vi "SVT Get Octave Value (N Ch).vi"(0 "octave spectra":T5(array[cluster]) {"band power" format="%.2f"; "nominal frequencies [Hz]" format="%.2f"}, 5 "frequency [Hz]":dbl=1000.0 format="%.2f", 9 "octave info":T1[](array[typedef]) {"engineering units" items=["custom..."=0, "V"=1, "A"=21, "C"=30, "pC"=31, "s"=32, "-"=29, "Pa"=2, "N"=20, "g"=3, "m/s^2"=4, "m/s"=5, "m"=6, "mm/s"=12, "mm"=13, "micron/s"=14, "micron"=15, "in/s^2"=7, "in/s"=8, "in"=9, "mil/s"=10, "mil"=11, "rad/s^2"=16, "rad/s"=17, "rad"=18, "deg/s^2"=26, "deg/s"=27, "deg"=28, "RPM"=22, "cycle/s^2"=23, "Hz"=24, "cycle"=25, "strain"=19]; "dB reference" format="%.2e"; "weighting filter" items=["Linear", "A-weighting", "B-weighting", "C-weighting", "ITU-R 468-4", "Dolby", "CCITT", "C-message", "Wb", "Wc", "Wd", "We", "Wf", "Wh", "Wj", "Wk", "Wm", "AES17 20 kHz lowpass", "AES17 40 kHz lowpass", "AES17 20 kHz highpass", "AES17 40 kHz highpass"]}, 11 "error in (no error)":errorcluster) -> (4 "band power values":dbl[](array[numeric]), 6 "unit labels":string[](array[string]), 8 "actual nominal frequencies [Hz]":dbl[](array[numeric]), 15 "error out":errorcluster)   [LabVIEW 2017, in "SoundVib_Octave_2014 standard.lvlib"]
doc: "Extracts the band power value of the <B>octave spectrum</B> at the specified input frequency. Finds the octave band that corresponds to the input frequency if the input frequency does not exactly coincide with a nominal frequency. Wire data to the <B>octave spectrum</B> input to determine the polymorphic instance to use or manually select the instance."
uses:
  <vilib>/addons/Sound and Vibration/svt_Octave/SoundVib_Octave_2014 standard.lvlib
  <vilib>/addons/_NISVFA/_Shared subVIs/Controls/svc_Octave Info.ctl
  <vilib>/addons/_NISVFA/_Shared subVIs/Controls/svc_Octave Standard.ctl
  <vilib>/addons/_NISVFA/_Shared subVIs/Controls/svc_Weighting Filter Text Ring.ctl
  <vilib>/addons/_NISVFA/_Shared subVIs/Controls/svc_Engineering Units Text Ring.ctl
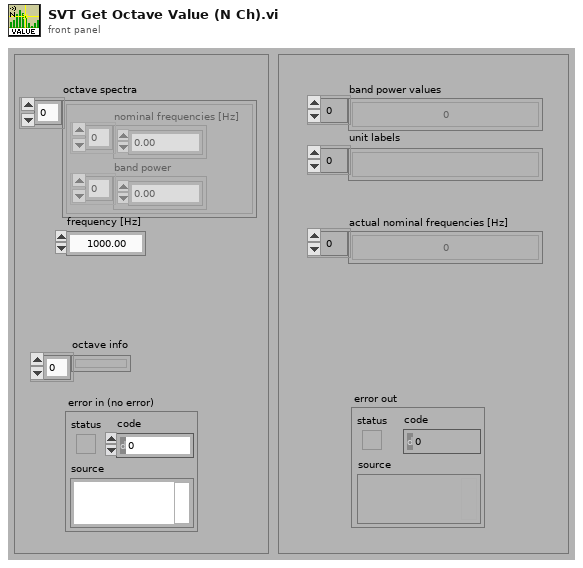
[diagram p1: front panel]
types:
  T1 = typedef "svc_Octave Info.ctl" = cluster{"standard":T2, "bandwidth":enum16{"1 octave", "1/3 octave", "1/6 octave", "1/12 octave", "1/24 octave"}, "low band":i32, "high band":i32, "weighting filter":T3, "dB reference":dbl, "dB On":bool, "unit label":string, "channel name":string, "description":string, "engineering units":T4, "custom label":string, "spectrum type":enum16{"power", "magnitude"}, "spectral density":bool, "filters settled":bool}
  T2 = typedef "svc_Octave Standard.ctl" = enum16{"ANSI S1.11", "IEC 61260"}
  T3 = typedef "svc_Weighting Filter Text Ring.ctl" = u16
  T4 = typedef "svc_Engineering Units Text Ring.ctl" = u16
  T5 = cluster{"nominal frequencies [Hz]":dbl[], "band power":dbl[]}[]
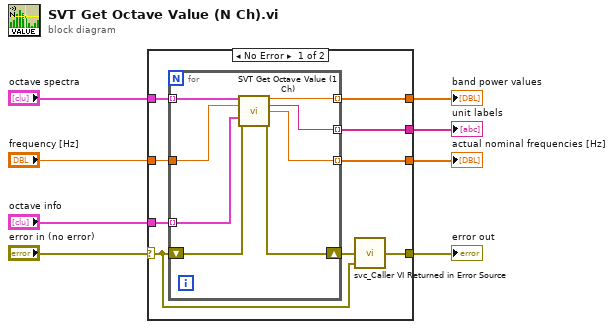
[diagram p0: block diagram]
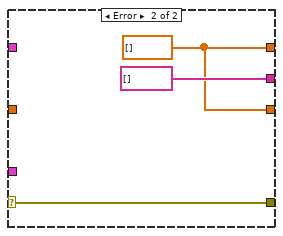
[diagram p2: hidden frame]
diagram:
  n1 = case shown="No Error" "error in (no error)" {
    tunnel: [w17 w28] -> w8
    tunnel: "octave info" -> [w15 _]
    tunnel: "octave spectra" -> [w16 _]
    tunnel: [w14 w26] -> w5
    tunnel: [w13 string[] []] -> w3
    tunnel: "frequency [Hz]" -> [w12 _]
    tunnel: [w11 w26] -> w2
    selector: "error in (no error)" -> [w9 w28]
    frame No Error {
      n2 = for {
        tunnel: w16 -> [w23] mode=indexing
        tunnel: w15 -> [w22] mode=indexing
        tunnel: [w21] -> w14 mode=indexing
        tunnel: [w20] -> w13 mode=indexing
        tunnel: w12 -> [w18]
        tunnel: [w19] -> w11 mode=indexing
        shift-right: [w24] -> w10
        shift-left: w9 -> [w25]
        n3 = call <vilib>:"SVT Get Octave Value (1 Ch).vi"("octave spectrum"=w23, "frequency [Hz]"=w18, "octave info"=w22, "error in (no error)"=w25) -> ("band power value"=w21:dbl, "unit label"=w20:string, "actual nominal frequency [Hz]"=w19:dbl, "error out"=w24:errorcluster)  [unwired: 8 in]
      }
      n4 = call <vilib>:"svc_Caller VI Returned in Error Source.vi"("warning input to caller"=w9, "error in (no error)"=w10) -> ("error out"=w17:errorcluster)  [unwired: 3 in]
    }
    frame Error {
      w26 = dbl[] [] ("Array")
    }
  }
  "error out" <- w8
  "band power values" <- w5
  "actual nominal frequencies [Hz]" <- w2
  "unit labels" <- w3
